vi "Camera.v7.vi"() -> ()   [LabVIEW 2015]
uses:
  Camera Properties.ctl
  Microscope Settings.ctl
  CameraState.ctl
  ModeEnum.ctl
  Stack_State.ctl
  Stack Track.ctl
  CameraControlTypeDef.ctl
  <vilib>/DAQmx/write.llb/DAQmx Write (Digital 1D Wfm NChan NSamp).vi
  <vilib>/DAQmx/write.llb/DAQmx Write (Analog 1D Wfm NChan NSamp).vi
  <vilib>/DAQmx/create/channels.llb/DAQmx Create Channel (DO-Digital Output).vi
  <vilib>/DAQmx/create/channels.llb/DAQmx Create Channel (AO-Voltage-Basic).vi
  <vilib>/Waveform/WDTOps.llb/WDT Number of Waveform Samples DBL.vi
  <vilib>/DAQmx/configure/timing.llb/DAQmx Timing (Sample Clock).vi
  <vilib>/Waveform/DWDTOps.llb/DWDT Uncompress Digital.vi
  <vilib>/DAQmx/miscellaneous.llb/DAQmx Fill In Error Info.vi
  <vilib>/vision/NI_Vision_Development_Module.lvlib
panel:
  out "Numeric 3":i32
  in  "Tab Control":enum32{"Camera Settings", "Recording"}(tab)
  in  "Microscope Settings":T1={"Mode"=enum."XY", {"Scanning Mode"=12.0, "Slit Width /%"=5.0}, "Piezo Position /um"=0.0, "Exposure/ms"=40.0, "Samples per millisecond"=100.0, "Relax/ms"=10.0, "Readout Direction"=2.0, "Trigger Source"=2.0, "Camera Delay"=11.0} {"Camera Delay" min=0.0 max=10.0 step=0.05; "Trigger Source" items=["Internal"=1.0, "External"=2.0]; "Readout Direction" items=["Forward"=1.0, "Backward"=2.0]; "?"."Scanning Mode" items=["Full Frame"=1.0, "Slit Scanning"=12.0]; "Piezo Position /um" min=0.0 max=10.0 step=0.1}
  in  "Scan":bool
  in  "Scan Continuously":bool
  out "error IO":errorcluster
  in  "V Height":dbl=2048.0 min=4.0 max=2048.0 step=4.0
  in  "V Offset":dbl min=0.0 max=0.0 step=4.0
  in  "H Offset":dbl min=0.0 max=0.0 step=4.0
  in  "H Width":dbl min=4.0 max=2048.0 step=4.0
  in  "Advanced DCAM Controls":i32(listbox) caption="Multicolumn Listbox"
  in  "Slit width":sgl
  in  "Properties":T2=4211904 items=["SENSOR MODE"=4212128, "CCD MODE"=4212384, "READOUT MODE"=4211872, "ACTIVE VIEW INDEX"=4343136, "BITS PER CHANNEL"=4342976, "IMAGE PIXEL TYPE"=4343296, "BINNING"=4215968, "EXPOSURE TIME"=2049184, "CONTRAST GAIN"=3163312, "CONTRAST OFFSET"=3163328, "LIGHT MODE"=2114720, "SENSITIVITY"=2114992, "PHOTON IMAGING MODE"=2115200, "HIGH DYNAMIC RANGE MODE"=3163360, "WHITE BALANCE"=3163568, "TEMPERATURE"=2115232, "TEMPERATURE TARGET"=2115264, "SENSOR COOLER FAN"=2115296, "LINEBUNDLE HEIGHT"=4212192, "MECHANICAL SHUTTER"=2115488, "BACK FOCUS POSITION"=8422304, "TRIGGER CONNECTOR"=1066432, "TRIGGER SOURCE"=1066144, "OUTPUT TRIGGER SOURCE"=1852576, "TRIGGER GLOBAL EXPOSURE"=2049680, "FIRST TRIGGER BEHAVIOR"=2049696, "CHANNEL SYNC"=1852352, "READOUT DIRECTION"=4211904, "PRE HSYNC COUNT"=1852704, "INTERNAL LINE SPEED"=4191408, "INTERNAL LINE INVERVAL"=4191424]
  out "Mixed Signal Graph":T3(graph)
  out "Image":T4(plugin-control)
  out "Histogram":T5(graph)
  in  "stop":bool
  in  "Signals Debugger":bool
  in  "Calibration":bool
  in  "MultiD Scan":bool
  in  "Stage Controller":bool
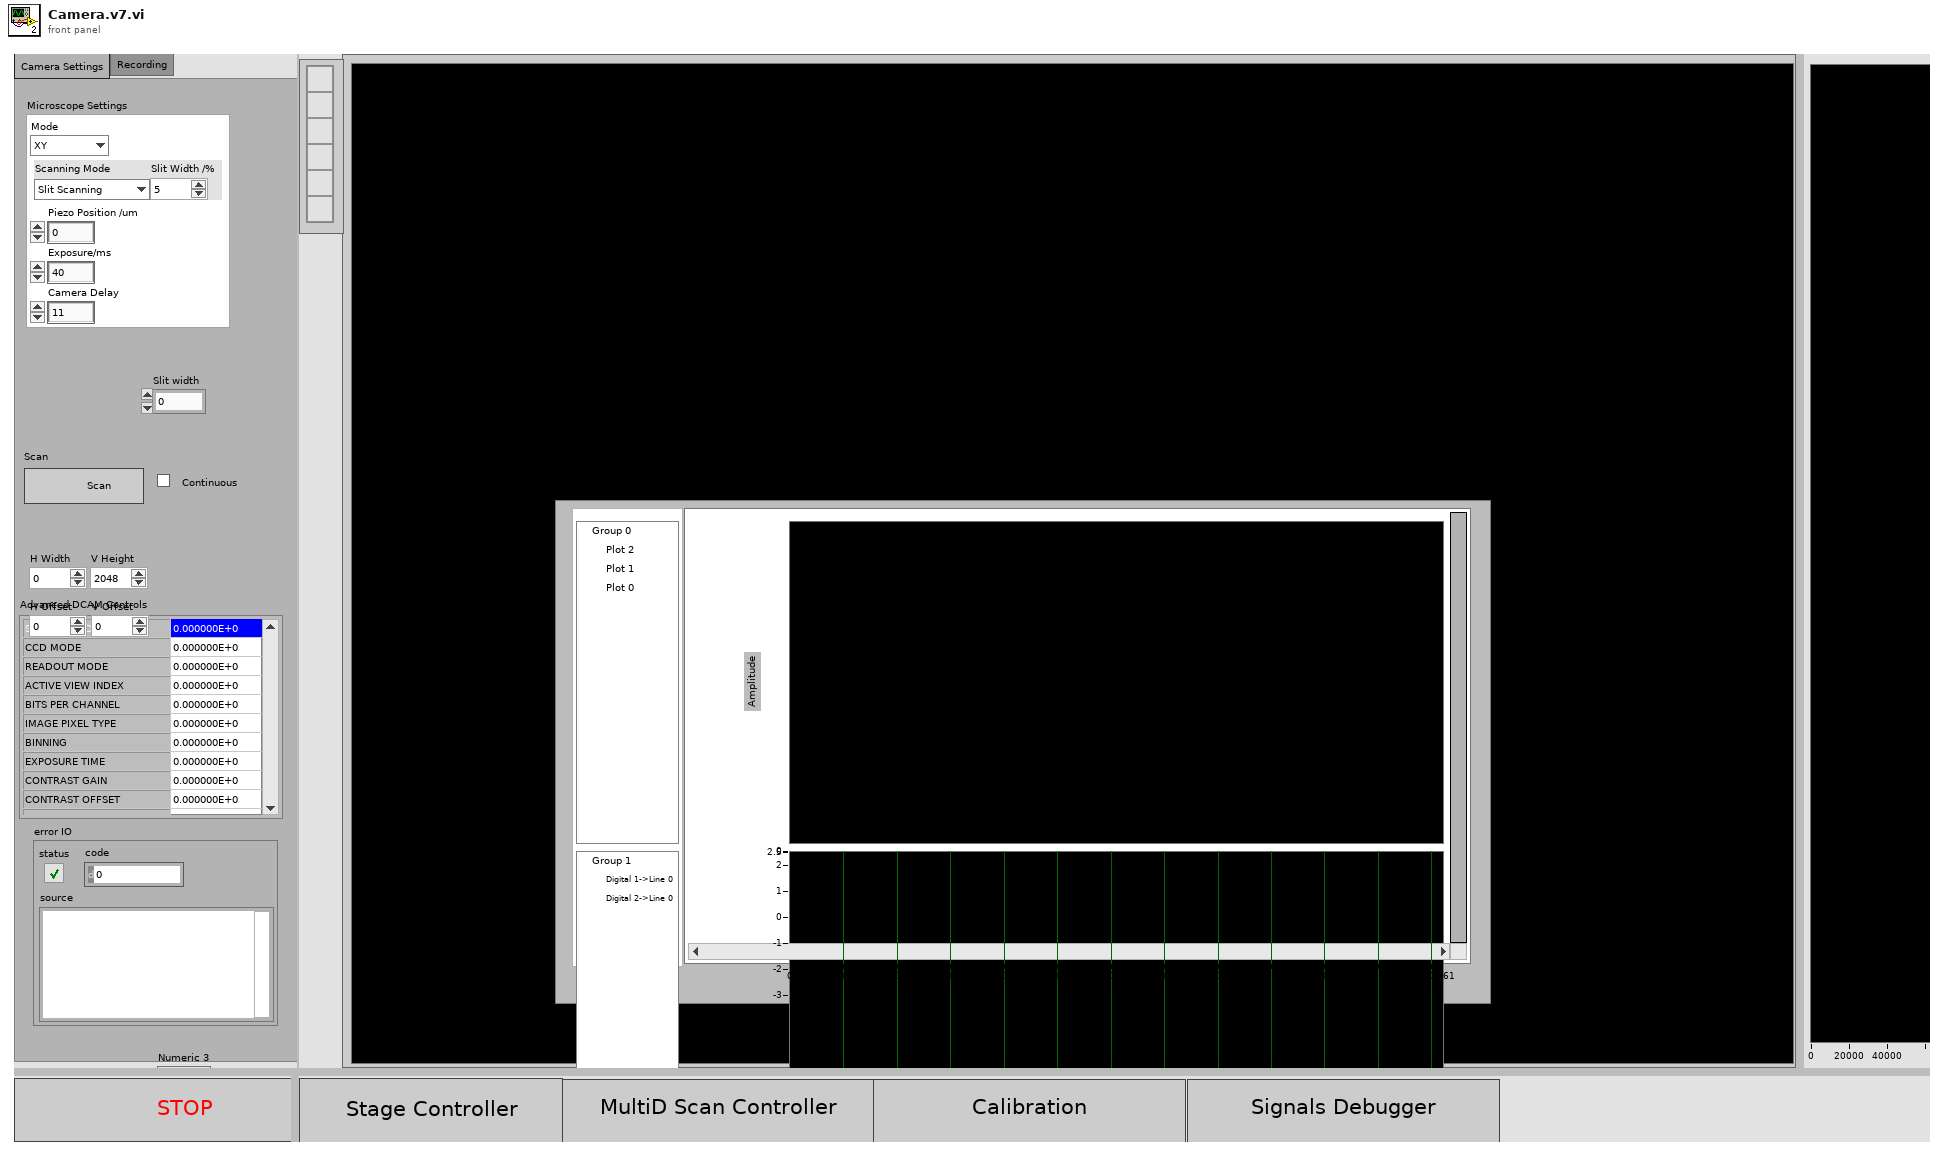
[diagram p1: front panel]
types:
  T1 = typedef "Microscope Settings.ctl" = cluster{"Mode":enum16{"X", "XY", "XYZ", "XYZT", "XYZC"}, cluster{"Scanning Mode":dbl, "Slit Width /%":dbl}, "Piezo Position /um":dbl, "Exposure/ms":dbl, "Samples per millisecond":dbl, "Relax/ms":dbl, "Readout Direction":dbl, "Trigger Source":dbl, "Camera Delay":dbl}
  T2 = typedef "Camera Properties.ctl" = u32
  T3 = cluster{waveform(dbl)[], "Digital Waveform":digitalwaveform, "Digital Waveform":digitalwaveform}
  T4 = typedef "IMAQ Image.ctl" = refnum<image>
  T5 = cluster{"Starting Value":sgl, "Incremental Value":sgl, "Histogram":u32[]}
  T6 = cluster{"height":u32, "width":u32, "datatype":u32}
  T7 = typedef "CameraState.ctl" = enum16{"init", "active", "deinit"}
  T8 = typedef "ModeEnum.ctl" = enum16{"Idle", "generateWaves", "runWaves", "stop"}
  T9 = cluster{"Mode":u32, "Polarity":u32, "Times":u32, "Delay":dbl}
  T10 = typedef "CameraControlTypeDef.ctl" = enum16{"Idle", "IntervalLineInt", "Ram Record", "HardDisk Record", "Disengage Update", "Update", "ROI", "Binning", "Scan Mode", "Trigger Mode", "Readout Mode", "Readout Direction", "Preview", "ROIWindow", "Trigger Source"}
  T11 = typedef "Stack_State.ctl" = cluster{"State":T12, "Stack Number":i32, "Image":u16[][], "Stacks":i32}
  T12 = typedef "Stack Track.ctl" = enum16{"Idle", "Display", "Start Sequence", "Read Disk", "STOP", "Collecting", "End"}
  T13 = typedef "Image Type" = u32
  T14 = cluster{"Value":i32, "Minimum":i32, "Maximum":i32, "Increment":i32}
  T15 = cluster{"State":T12, "Timeout":i32, "Data 16":u16[][], "Timeout":i32}
  T16 = cluster{"Enum":T10, "Trigger Source":dbl, "timeout in ms (-1)":i32}
  T17 = cluster{"Enum":T10, "Trigger Source":dbl, "Property ID":u32}
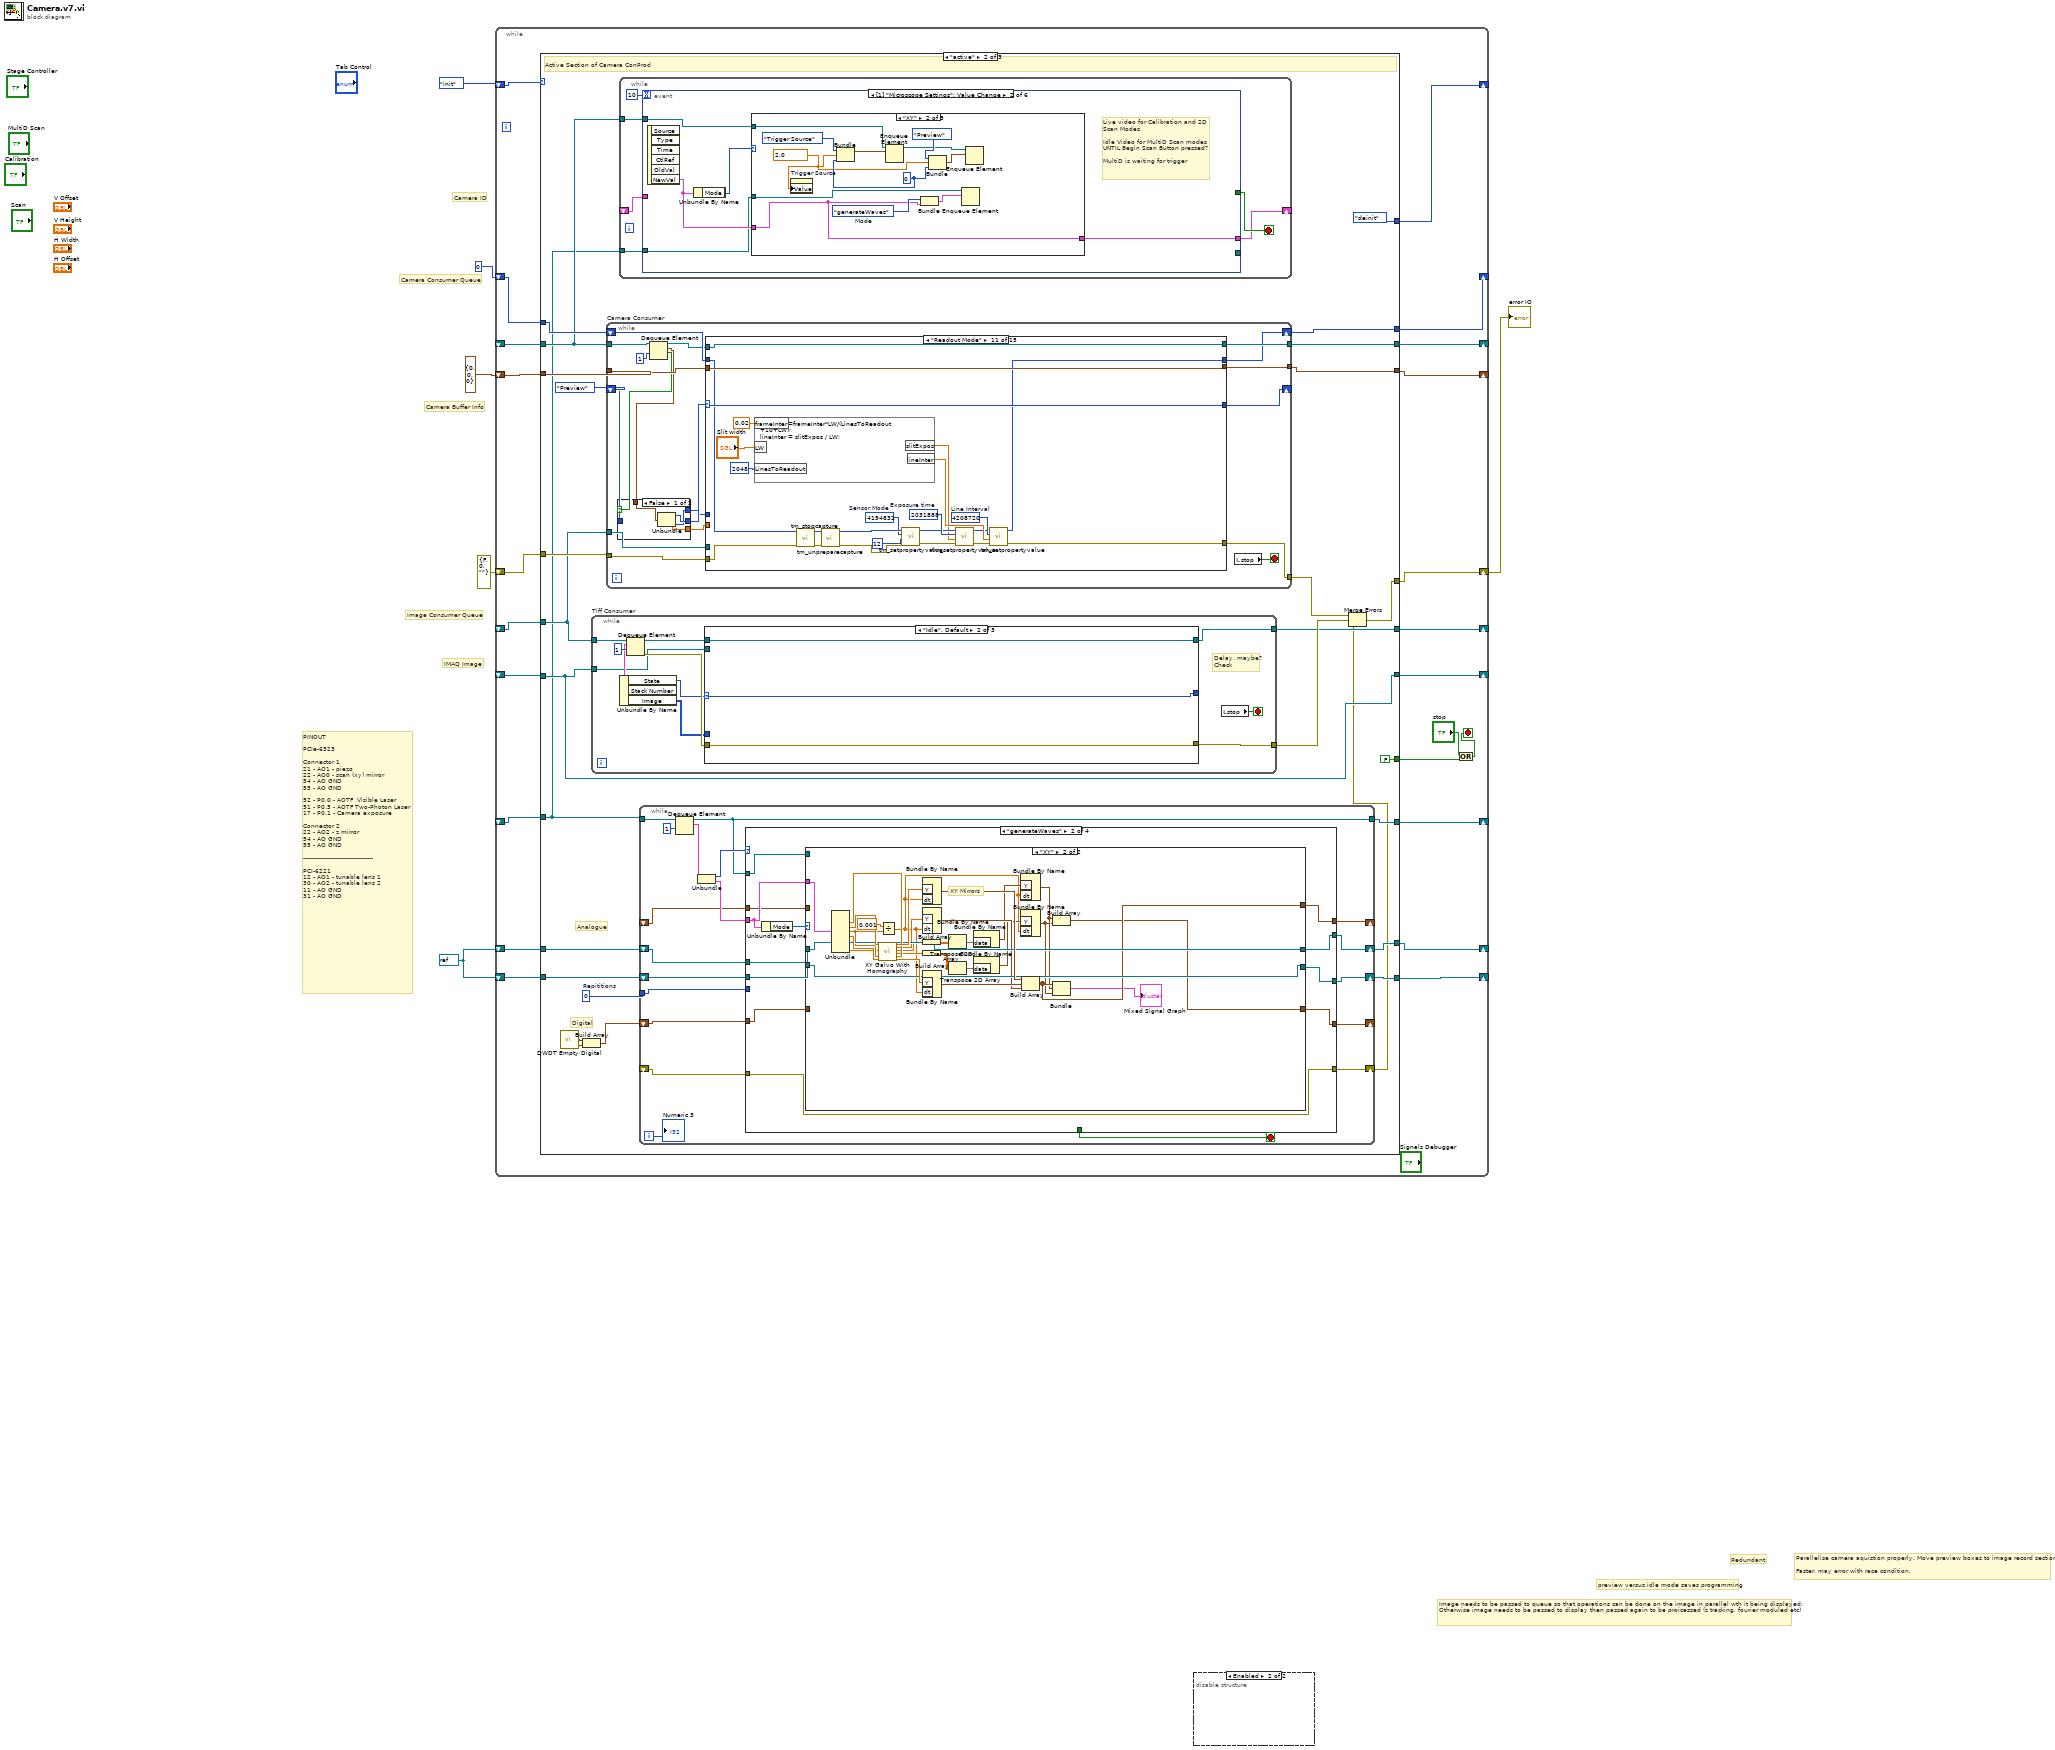
[diagram p0: block diagram]
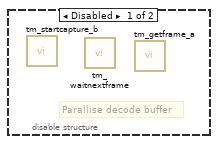
[diagram p2: hidden frame]
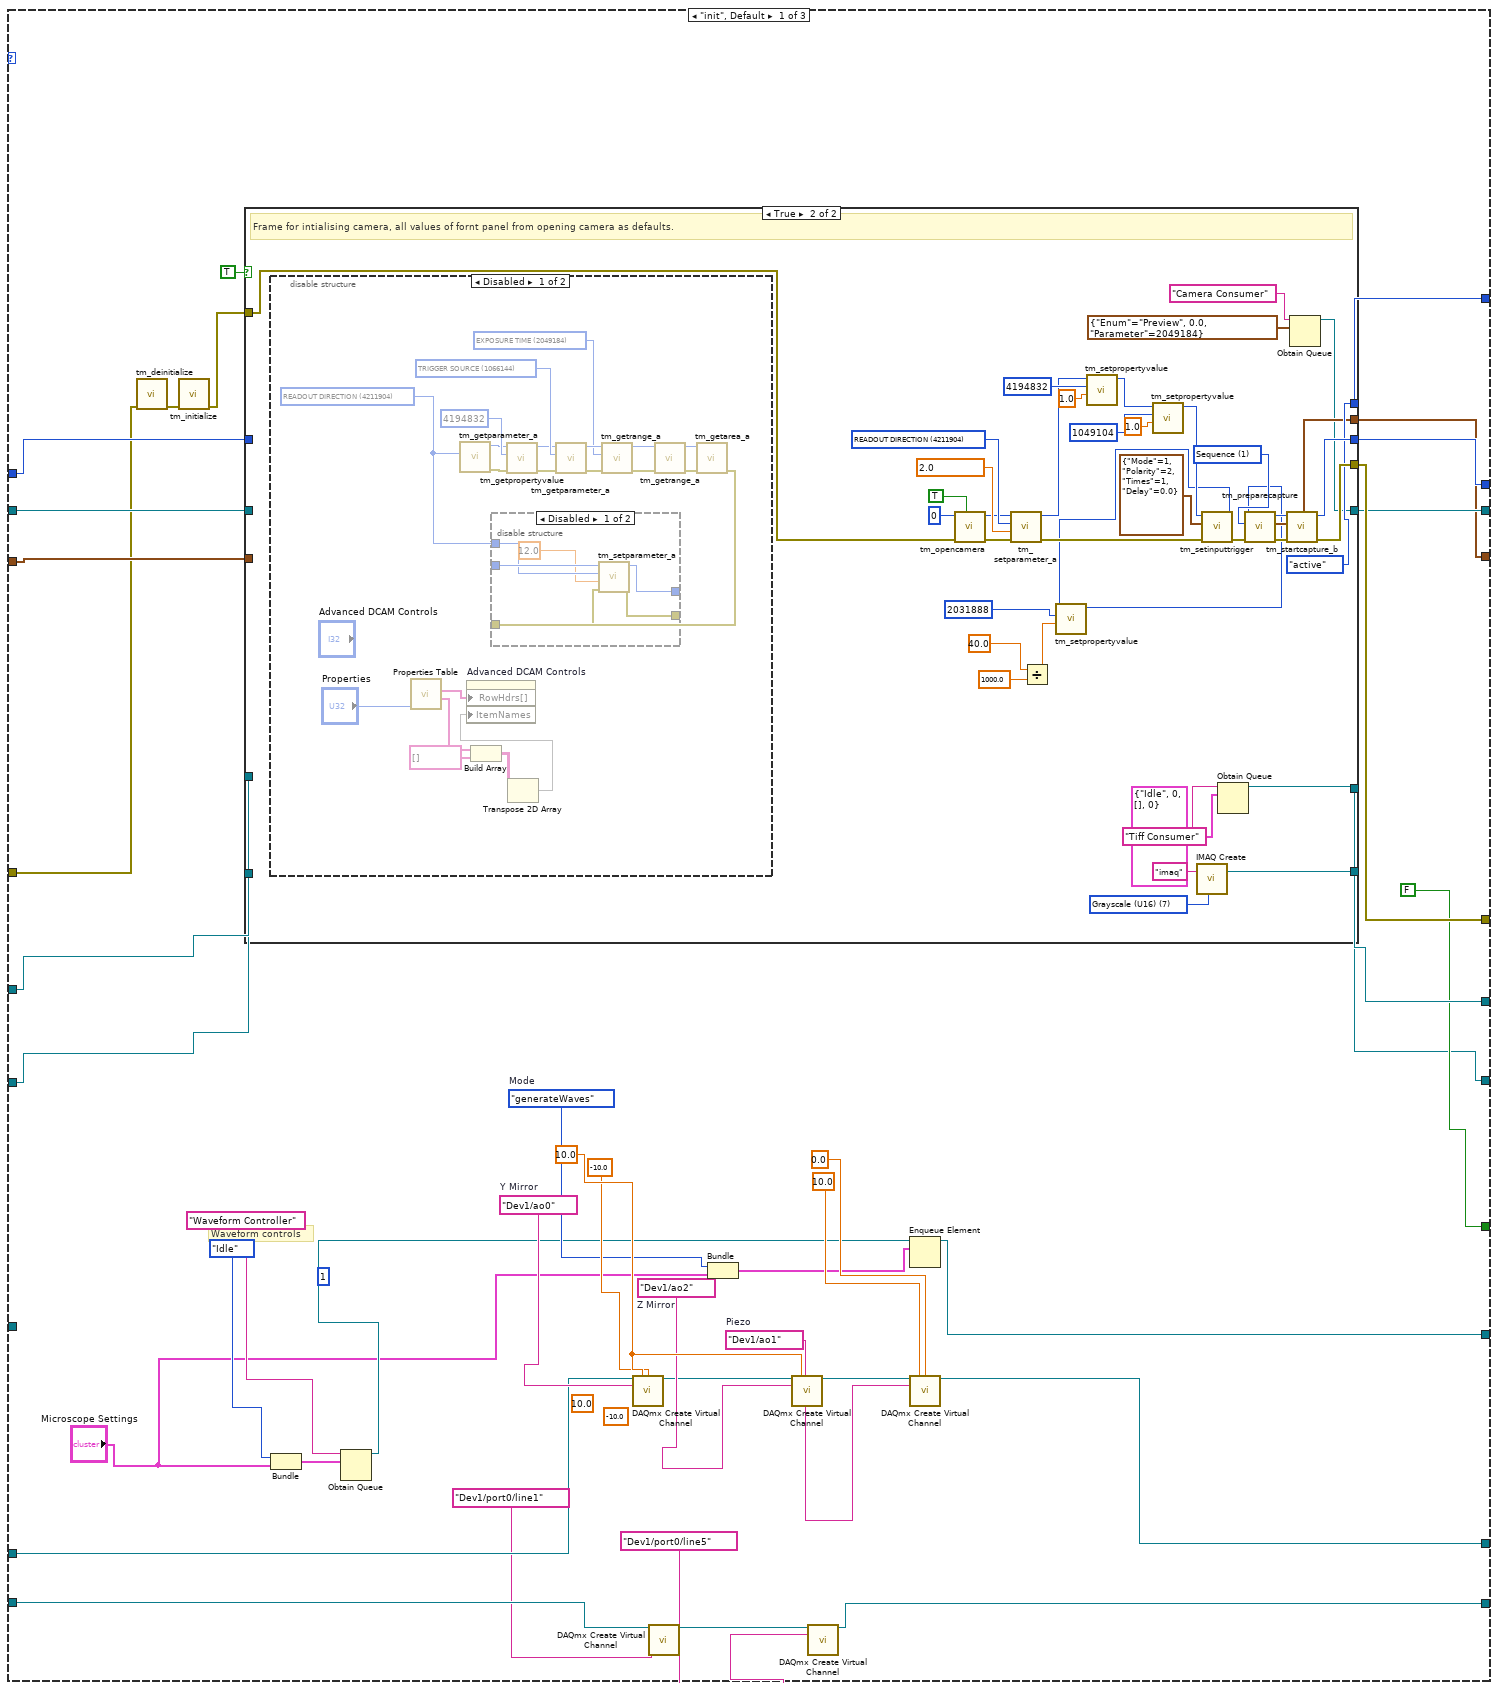
[diagram p3: hidden frame]
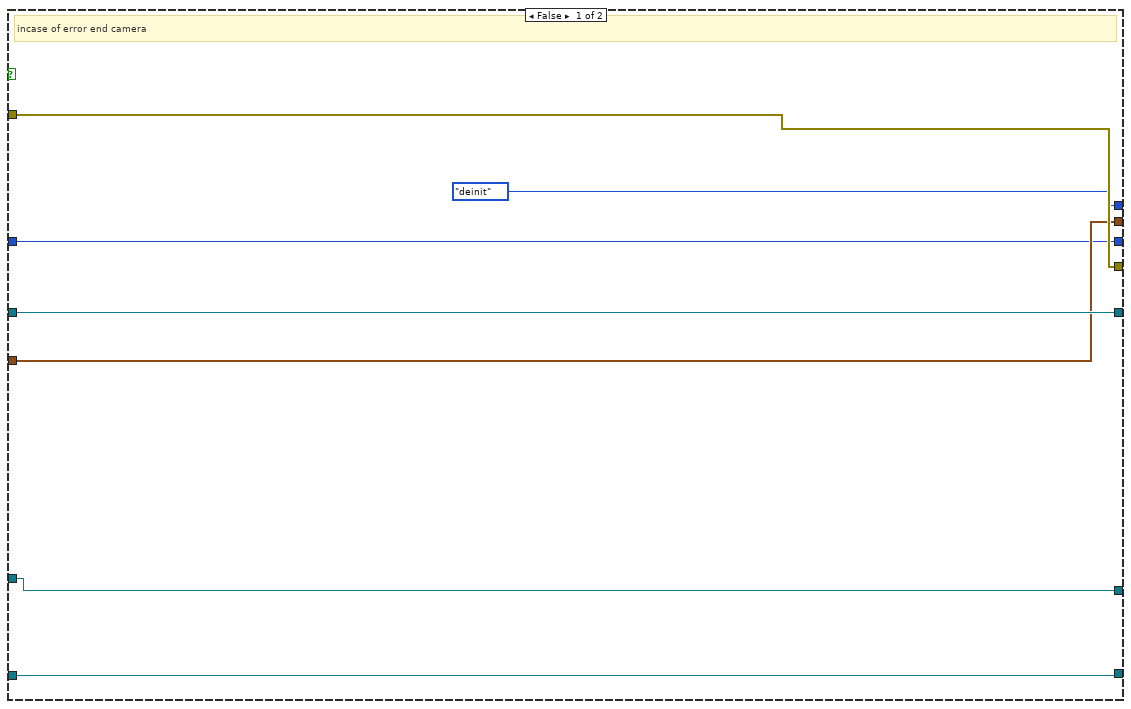
[diagram p4: hidden frame]
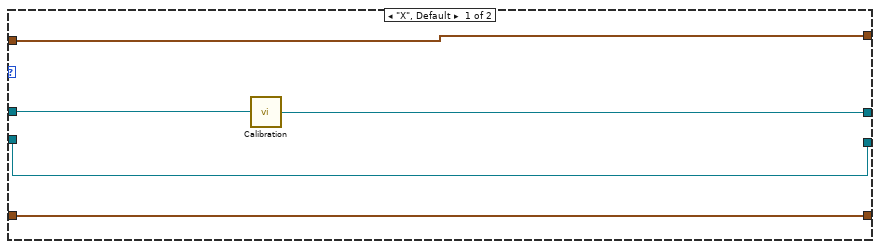
[diagram p8: hidden frame]
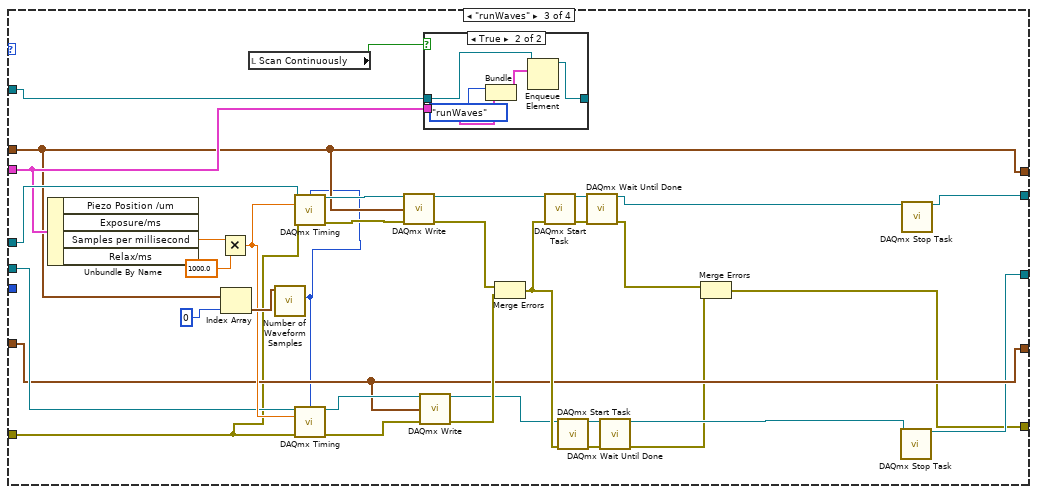
[diagram p9: hidden frame]
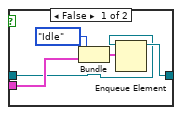
[diagram p10: hidden frame]
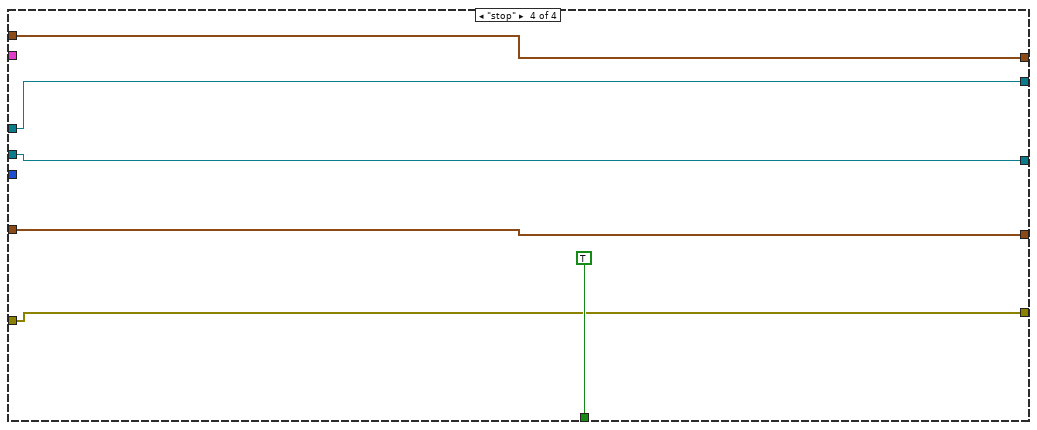
[diagram p11: hidden frame]
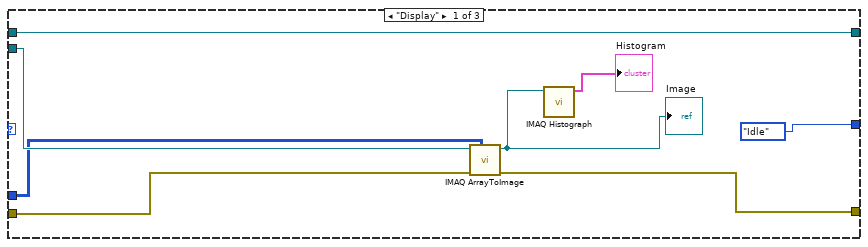
[diagram p12: hidden frame]
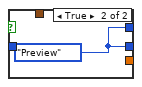
[diagram p14: hidden frame]
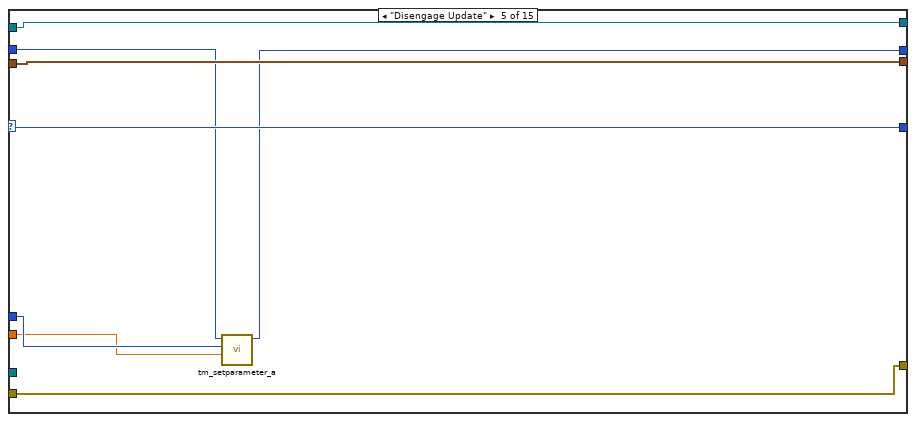
[diagram p19: hidden frame]
diagram:
  w3 = refnum<k21> refnum ("Mirror Z 2")
  # "PINOUT\n\nPCIe-6323\n\nConnector 1\n21 - AO1 - piezo\n22 - AO0 - scan (xy) mirror\n54 - AO GND\n55 - AO GND\n\n52 - P0.0 - AOTF  Visible Laser\n51 - P0.5 - AOTF Two-Photon Laser\n17 - P0.1 - Camera exposure\n\nConnector 2\n22 - AO2 - z mirror\n54 - AO GND\n55 - AO GND\n\n-----------------------------------\n\nPCI-6221\n12 - AO1 - tunable lens 1\n30 - AO2 - tunable lens 2\n11 - AO GND\n31 - AO GND"
  # "IMAQ Image"
  # "Camera Buffer Info"
  # "Image needs to be passed to queue so that operations can be done on the image in parallel wth it being displayed;\nOtherwise image needs to be passed to display then passed again to be proicessed (z tracking, fourier moduled etc)"
  # "preview versus idle mode saves programming"
  # "Parallelise camera aquistion properly. Move preview boxes to image record section.\n\nFaster. may error with race condition."
  # "Redundant"
  # "Image Consumer Queue"
  # "Camera Consumer Queue"
  # "Camera ID"
  n1 = while {
    shift-right: [w29] -> _
    shift-left: CameraState."init" -> [w28]
    shift-right: [w27] -> _
    shift-left: u32 0 ("Handle out") -> [w26]
    shift-right: [w25] -> w5
    shift-left: errorcluster {"status"=FALSE, "code"=0, "source"=""} ("error IO") -> [w24]
    shift-right: [w22] -> _
    shift-left: _ -> [w21]
    shift-right: [w23] -> _
    shift-left: _ -> [w20]
    shift-right: [w16] -> _
    shift-left: T6 {"height"=0, "width"=0, "datatype"=0} ("Buffer Info") -> [w15]
    shift-right: [w14] -> _
    shift-left: _ -> [w13]
    shift-right: [w12] -> _
    shift-left: w3 -> [w11]
    shift-right: [w9] -> _
    shift-left: w3 -> [w10]
    shift-right: [w8] -> _
    shift-left: _ -> [w7]
    stop <- w18 stop-if-true
    n2 = case shown="\"active\"" w28 {
      tunnel: [w68 CameraState."deinit" CameraState."init"] -> w29
      tunnel: [w67 w170 w561] -> w27
      tunnel: w26 -> [w45 w171 w561]
      tunnel: [w66 w169 w564] -> w25
      tunnel: w24 -> [w44 w163 w565]
      tunnel: [w65 w166 w548] -> w23
      tunnel: [w64 w165 w544] -> w22
      tunnel: w21 -> [w62 w158 w544]
      tunnel: w20 -> [w63 w156 w548]
      tunnel: [FALSE ("stop") FALSE ("stop") TRUE ("stop")] -> w17
      tunnel: [w60 w161 w558] -> w16
      tunnel: w15 -> [w59 w160 w558]
      tunnel: w13 -> [w57 w157 w557]
      tunnel: [w58 w157 w557] -> w14
      tunnel: w7 -> [_ w148 w543]
      tunnel: [w49 w149 w555] -> w12
      tunnel: w11 -> [w46 w152 w555]
      tunnel: w10 -> [w42 w151 w553]
      tunnel: [w33 w150 w553] -> w9
      tunnel: [w41 w147 w543] -> w8
      frame "init", Default {
        (unwired) 1 ("max queue size (-1, unlimited)")
        w39 = ModeEnum."generateWaves"  # Mode
        (unwired) -10.0 ("minimum value")
        (unwired) 10.0 ("maximum value")
        w52 = tag "Dev1/ao1"  # Piezo
        w53 = tag "Dev1/ao2"  # Z Mirror
        w54 = tag "Dev1/ao0"  # Y Mirror
        w56 = 10.0 ("maximum value")
        # "Waveform controls"
        n3 = call "tm_deinitialize.vi"("error in (no error)"=w44) -> ("error out"=w70:errorcluster)  [unwired: 10 in]
        n4 = call "tm_initialize.vi"("error in (no error)"=w70) -> ("error out"=w69:errorcluster)  [unwired: 7 in, 3 out]
        n5 = case shown="True" TRUE {
          tunnel: w69 -> [w77 w114]
          tunnel: [CameraState."deinit" CameraState."active"] -> w68
          tunnel: [w77 w111] -> w66
          tunnel: [w72 w109] -> w67
          tunnel: [w75 w98] -> w65
          tunnel: [w74 w106] -> w64
          tunnel: w63 -> [w75 _]
          tunnel: w62 -> [w74 _]
          tunnel: [w73 w104] -> w60
          tunnel: w59 -> [w73 _]
          tunnel: w45 -> [w72 _]
          tunnel: [w71 w101] -> w58
          tunnel: w57 -> [w71 _]
          frame False {
            # "incase of error end camera"
          }
          frame True {
            w96 = sgl 2.0 items=["Forward"=1.0, "Backward"=2.0] ("Readout Direction")
            w97 = u32 4211904 items=["SENSOR MODE"=4212128, "CCD MODE"=4212384, "READOUT MODE"=4211872, "ACTIVE VIEW INDEX"=4343136, "BITS PER CHANNEL"=4342976, "IMAGE PIXEL TYPE"=4343296, "BINNING"=4215968, "EXPOSURE TIME"=2049184, "CONTRAST GAIN"=3163312, "CONTRAST OFFSET"=3163328, "LIGHT MODE"=2114720, "SENSITIVITY"=2114992, "PHOTON IMAGING MODE"=2115200, "HIGH DYNAMIC RANGE MODE"=3163360, "WHITE BALANCE"=3163568, "TEMPERATURE"=2115232, "TEMPERATURE TARGET"=2115264, "SENSOR COOLER FAN"=2115296, "LINEBUNDLE HEIGHT"=4212192, "MECHANICAL SHUTTER"=2115488, "BACK FOCUS POSITION"=8422304, "TRIGGER CONNECTOR"=1066432, "TRIGGER SOURCE"=1066144, "OUTPUT TRIGGER SOURCE"=1852576, "TRIGGER GLOBAL EXPOSURE"=2049680, "FIRST TRIGGER BEHAVIOR"=2049696, "CHANNEL SYNC"=1852352, "READOUT DIRECTION"=4211904, "PRE HSYNC COUNT"=1852704, "INTERNAL LINE SPEED"=4226000, "INTERNAL LINE INTERVAL"=4226016] ("Parameter")
            w103 = T13 7 items=["Grayscale (U8)", "Grayscale (I16)", "Grayscale (SGL)", "Complex (CSG)", "RGB (U32)", "HSL (U32)", "RGB (U64)", "Grayscale (U16)"] ("Image Type")
            w113 = 1 items=["Snap", "Sequence"] ("Capture mode")
            # "Frame for intialising camera, all values of fornt panel from opening camera as defaults."
            n6 = disable-structure shown="Disabled" {
              frame Disabled {
                w135 = u32 2049184 items=["SENSOR MODE"=4212128, "CCD MODE"=4212384, "READOUT MODE"=4211872, "ACTIVE VIEW INDEX"=4343136, "BITS PER CHANNEL"=4342976, "IMAGE PIXEL TYPE"=4343296, "BINNING"=4215968, "EXPOSURE TIME"=2049184, "CONTRAST GAIN"=3163312, "CONTRAST OFFSET"=3163328, "LIGHT MODE"=2114720, "SENSITIVITY"=2114992, "PHOTON IMAGING MODE"=2115200, "HIGH DYNAMIC RANGE MODE"=3163360, "WHITE BALANCE"=3163568, "TEMPERATURE"=2115232, "TEMPERATURE TARGET"=2115264, "SENSOR COOLER FAN"=2115296, "LINEBUNDLE HEIGHT"=4212192, "MECHANICAL SHUTTER"=2115488, "BACK FOCUS POSITION"=8422304, "TRIGGER CONNECTOR"=1066432, "TRIGGER SOURCE"=1066144, "OUTPUT TRIGGER SOURCE"=1852576, "TRIGGER GLOBAL EXPOSURE"=2049680, "FIRST TRIGGER BEHAVIOR"=2049696, "CHANNEL SYNC"=1852352, "READOUT DIRECTION"=4211904, "PRE HSYNC COUNT"=1852704, "INTERNAL LINE SPEED"=4191408, "INTERNAL LINE INVERVAL"=4191424] ("Parameter")
                w118 = T2 4211904 items=["SENSOR MODE"=4212128, "CCD MODE"=4212384, "READOUT MODE"=4211872, "ACTIVE VIEW INDEX"=4343136, "BITS PER CHANNEL"=4342976, "IMAGE PIXEL TYPE"=4343296, "BINNING"=4215968, "EXPOSURE TIME"=2049184, "CONTRAST GAIN"=3163312, "CONTRAST OFFSET"=3163328, "LIGHT MODE"=2114720, "SENSITIVITY"=2114992, "PHOTON IMAGING MODE"=2115200, "HIGH DYNAMIC RANGE MODE"=3163360, "WHITE BALANCE"=3163568, "TEMPERATURE"=2115232, "TEMPERATURE TARGET"=2115264, "SENSOR COOLER FAN"=2115296, "LINEBUNDLE HEIGHT"=4212192, "MECHANICAL SHUTTER"=2115488, "BACK FOCUS POSITION"=8422304, "TRIGGER CONNECTOR"=1066432, "TRIGGER SOURCE"=1066144, "OUTPUT TRIGGER SOURCE"=1852576, "TRIGGER GLOBAL EXPOSURE"=2049680, "FIRST TRIGGER BEHAVIOR"=2049696, "CHANNEL SYNC"=1852352, "READOUT DIRECTION"=4211904, "PRE HSYNC COUNT"=1852704, "INTERNAL LINE SPEED"=4191408, "INTERNAL LINE INVERVAL"=4191424] ("Parameter")
                w138 = u32 1066144 items=["SENSOR MODE"=4212128, "CCD MODE"=4212384, "READOUT MODE"=4211872, "ACTIVE VIEW INDEX"=4343136, "BITS PER CHANNEL"=4342976, "IMAGE PIXEL TYPE"=4343296, "BINNING"=4215968, "EXPOSURE TIME"=2049184, "CONTRAST GAIN"=3163312, "CONTRAST OFFSET"=3163328, "LIGHT MODE"=2114720, "SENSITIVITY"=2114992, "PHOTON IMAGING MODE"=2115200, "HIGH DYNAMIC RANGE MODE"=3163360, "WHITE BALANCE"=3163568, "TEMPERATURE"=2115232, "TEMPERATURE TARGET"=2115264, "SENSOR COOLER FAN"=2115296, "LINEBUNDLE HEIGHT"=4212192, "MECHANICAL SHUTTER"=2115488, "BACK FOCUS POSITION"=8422304, "TRIGGER CONNECTOR"=1066432, "TRIGGER SOURCE"=1066144, "OUTPUT TRIGGER SOURCE"=1852576, "TRIGGER GLOBAL EXPOSURE"=2049680, "FIRST TRIGGER BEHAVIOR"=2049696, "CHANNEL SYNC"=1852352, "READOUT DIRECTION"=4211904, "PRE HSYNC COUNT"=1852704, "INTERNAL LINE SPEED"=4191408, "INTERNAL LINE INVERVAL"=4191424] ("Parameter")
                n7 = call "Properties Table.vi"("Properties"="Properties") -> ("Value Stirngs Out"=w123:string[], "Row Headers"=w124:string[])  [unwired: 4 in, 2 out]
                n8 = call "tm_getparameter_a.vi"("Parameter"=w118) -> ("error out"=w127:errorcluster, "Handle out"=w129:u32)  [unwired: 8 in, 1 out]
                n9 = Build Array(w123, string[] [] ("element")) -> (w121:string[][])
                n10 = call "tm_getpropertyvalue.vi"("error in (no error)"=w127, "Property ID"=u32 4194832, "Handle in"=w129) -> ("error out"=w128:errorcluster, "Handle out"=w117:u32)  [unwired: 6 in, 1 out]
                n11 = Transpose 2D Array(2D array=w121) -> (transposed array=w120:string[][])
                n12 = property on="Advanced DCAM Controls" class="MCListbox (strict)"("RowHdrs[]"=w124, "ItemNames"=w120) -> ()  [unwired: 2 in, 2 out]
                n13 = call "tm_getparameter_a.vi"("error in (no error)"=w128, "Parameter"=w138, "Handle in"=w117) -> ("error out"=w136:errorcluster, "Handle out"=w137:u32)  [unwired: 6 in, 1 out]
                n14 = call "tm_getrange_a.vi"("error in (no error)"=w136, "Parameter"=w135, "Handle in"=w137) -> ("error out"=w133:errorcluster, "Handle out"=w134:u32)  [unwired: 2 in, 5 out]
                n15 = call "tm_getrange_a.vi"("error in (no error)"=w133, "Handle in"=w134) -> ("error out"=w132:errorcluster, "Handle out"=w131:u32)  [unwired: 3 in, 5 out]
                n16 = call "tm_getarea_a.vi"("error in (no error)"=w132, "Handle in"=w131) -> ("error out"=w119:errorcluster, "H Offset"=w126:T14)  [unwired: 4 in, 4 out]
                n17 = disable-structure shown="Disabled" {
                  disable-tunnel: _ -> [w144 _]
                  disable-tunnel: [w143 _] -> _
                  disable-tunnel: w119 -> [w142 w145]
                  disable-tunnel: [w141 w145] -> _
                  disable-tunnel: w118 -> [w140 _]
                  frame Disabled {
                    n18 = call "tm_setparameter_a.vi"("error in (no error)"=w142, "Value in"=12.0, "Parameter"=w140, "Handle in"=w144) -> ("error out"=w141:errorcluster, "Handle out"=w143:u32)  [unwired: 6 in]
                  }
                  frame Enabled {
                  }
                }
              }
              frame Enabled {
              }
            }
            n19 = call "tm_opencamera.vi"("Force Open"=TRUE, "error in (no error)"=w114, "Camera Index"=u32 0) -> ("error out"=w94:errorcluster, "Handle out"=w95:u32)  [unwired: 6 in, 1 out]
            n20 = call "tm_setparameter_a.vi"("error in (no error)"=w94, "Value in"=w96, "Parameter"=w97, "Handle in"=w95) -> ("error out"=w85:errorcluster, "Handle out"=w84:u32)  [unwired: 6 in]
            n21 = Divide(x=sgl 40.0 ("Value in"), y=sgl 1000.0) -> (x/y=w78:sgl)
            n22 = call "tm_setpropertyvalue.vi"("Value in"=sgl 1.0, "Property ID"=u32 4194832, "Handle in"=w84) -> ("Handle out"=w88:u32)  [unwired: 7 in, 1 out]
            n23 = call "tm_setpropertyvalue.vi"("Value in"=sgl 1.0, "Property ID"=u32 1049104, "Handle in"=w88) -> ("Handle out"=w86:u32)  [unwired: 7 in, 1 out]
            n24 = call "IMAQ Create"("Image Name"="imaq", "Image Type"=w103) -> ("New Image"=w101:T4)  [unwired: 3 in, 1 out]
            n25 = call <userlib>:"tm_setinputtrigger.vi"("error in (no error)"=w85, "Parameters"=T9 {"Mode"=1, "Polarity"=2, "Times"=1, "Delay"=0.0}, "Handle in"=w86) -> ("error out"=w93:errorcluster, "Handle out"=w82:u32)  [unwired: 7 in]
            n26 = call "tm_setpropertyvalue.vi"("Value in"=w78, "Property ID"=u32 2031888, "Handle in"=w82) -> ("Handle out"=w81:u32)  [unwired: 7 in, 1 out]
            n27 = Obtain Queue(name (unnamed)="Tiff Consumer", element data type=T11 {"State"=enum."Idle", "Stack Number"=0, "Image"=[], "Stacks"=0} ("input cluster")) -> (queue out=w106:refnum<queue>)  [unwired: 3 in, 2 out]
            n28 = call "tm_preparecapture.vi"("error in (no error)"=w93, "Capture mode"=w113, "Handle in"=w81) -> ("error out"=w112:errorcluster, "Buffer Info"=w104:T6, "Handle out"=w110:u32)  [unwired: 5 in, 1 out]
            n29 = call "tm_startcapture_b.vi"("error in (no error)"=w112, "Handle in"=w110) -> ("error out"=w111:errorcluster, "Handle out"=w109:u32)  [unwired: 8 in]
            n30 = Obtain Queue(name (unnamed)="Camera Consumer", element data type=cluster{"Enum":T10, dbl, "Parameter":u32} {"Enum"=enum."Preview", 0.0, "Parameter"=2049184}) -> (queue out=w98:refnum<queue>)  [unwired: 3 in, 2 out]
          }
        }
        n31 = Bundle("Mode"=ModeEnum."Idle", "Microscope Settings"="Microscope Settings") -> (w36:cluster{"Mode":T8, "Microscope Settings":T1})  [unwired: 1 in]
        n32 = Obtain Queue(name (unnamed)="Waveform Controller", element data type=w36) -> (queue out=w35:refnum<queue>)  [unwired: 3 in, 2 out]
        n33 = call-poly <vilib>:"DAQmx Create Virtual Channel.vi"("task in"=w46, "maximum value"=w56, "minimum value"=-10.0, "physical channels"=w54) -> ("task out"=w48:refnum<k21>)  [unwired: 10 in, 1 out]
        n34 = call-poly <vilib>:"DAQmx Create Virtual Channel.vi"("task in"=w42, "lines"=tag "Dev1/port0/line1") -> ("task out"=w43:refnum<k21>)  [unwired: 12 in, 1 out]
        n35 = Bundle("Mode"=w39, "Microscope Settings"="Microscope Settings") -> (w40:cluster{"Mode":T8, "Microscope Settings":T1})  [unwired: 1 in]
        n36 = call-poly <vilib>:"DAQmx Create Virtual Channel.vi"("task in"=w48, "maximum value"=w56, "physical channels"=w53) -> ("task out"=w47:refnum<k21>)  [unwired: 11 in, 1 out]
        n37 = call-poly <vilib>:"DAQmx Create Virtual Channel.vi"("task in"=w43, "lines"=tag "Dev1/port0/line5") -> ("task out"=w33:refnum<k21>)  [unwired: 12 in, 1 out]
        n38 = Enqueue Element(queue=w35, element=w40) -> (queue out=w41:refnum<queue>)  [unwired: 2 in, 2 out]
        n39 = call-poly <vilib>:"DAQmx Create Virtual Channel.vi"("task in"=w47, "maximum value"=10.0 ("minimum value"), "minimum value"=0.0 ("maximum value"), "physical channels"=w52) -> ("task out"=w49:refnum<k21>)  [unwired: 10 in, 1 out]
      }
      frame "active" {
        w155 = 0  # Repititions
        # "Digital"
        # "Analogue"
        # "Active Section of Camera ConProd"
        n40 = call <vilib>:"DWDT Empty Digital.vi"() -> ("digital waveform out"=w153:digitalwaveform)  [unwired: 5 in]
        n41 = Build Array(w153, w153) -> (w154:digitalwaveform[])
        n42 = while "Tiff Consumer" {
          tunnel: [w295] -> w168
          tunnel: [w298] -> w165
          tunnel: w158 -> [w300]
          tunnel: w157 -> [w292]
          stop <- w302 stop-if-true
          # "Delay, maybe?\nCheck"
          n43 = Dequeue Element(queue=w300, timeout in ms (-1)=1) -> (queue out=w297:refnum<queue>, element=w299:T11, error out=w296:errorcluster)  [unwired: 1 in, 1 out]
          n44 = Unbundle By Name(w299) -> ("State"=w293:T12, "Image"=w294:u16[][])  [unwired: 1 out]
          n45 = case shown="\"Idle\", Default" w293 {
            selector: w293 -> [_ w313 w314]
            tunnel: [w310 w312 w315] -> w298
            tunnel: w297 -> [w310 w312 w315]
            tunnel: [Stack_Track."Idle" ("State") w313 w314] -> _
            tunnel: w294 -> [w305 _ _]
            tunnel: w292 -> [w309 _ _]
            tunnel: w296 -> [w308 w311 w316]
            tunnel: [w307 w311 w316] -> w295
            frame "Display" {
              n46 = call "IMAQ ArrayToImage"("Image Pixels (U16)"=w305, "error in (no error)"=w308, "Image"=w309) -> ("error out"=w307:errorcluster, "Image Out"=w304:T4)  [unwired: 7 in]
              "Image" <- w304
              n47 = call "IMAQ Histograph"("Image"=w304) -> ("Histogram Graph"=→"Histogram":T5)  [unwired: 7 in, 3 out]
            }
            frame "Idle", Default {
            }
            frame "Start Sequence" {
            }
          }
          n48 = local read "stop"() -> (w302:bool)
        }
        n49 = while "Camera Consumer" {
          tunnel: w163 -> [w334]
          tunnel: [w318] -> w167
          tunnel: w156 -> [w327]
          tunnel: [w335] -> w166
          shift-right: [w333] -> _
          shift-left: CameraControlTypeDef."Preview" ("Enum") -> [w323]
          tunnel: [w330] -> w161
          tunnel: w160 -> [w329]
          tunnel: w158 -> [w322]
          shift-right: [w331] -> w170
          shift-left: w171 -> [w332]
          stop <- w317 stop-if-true
          n50 = Dequeue Element(queue=w327, timeout in ms (-1)=1) -> (queue out=w326:refnum<queue>, element=w321:cluster{"Enum":T10, dbl, "Parameter":u32}, timed out?=w325:bool)  [unwired: 1 in, 1 out]
          n51 = case shown="False" w325 {
            tunnel: [w338 w340] -> w324
            tunnel: w323 -> [_ _]
            tunnel: w321 -> [w339 _]
            tunnel: [w337 _] -> w320
            tunnel: [w336 w340] -> w319
            frame False {
              n52 = Unbundle(w339) -> ("Enum"=w338:T10, w337:dbl, "Parameter"=w336:u32)
            }
            frame True {
              w340 = CameraControlTypeDef."Preview" ("Enum")
            }
          }
          n53 = case shown="\"Readout Mode\"" w324 {
            selector: w324 -> [w344 w349 w354 w359 w367 w372 w377 w382 w387 w392 w416 w422 _ w451 _]
            tunnel: w326 -> [w343 w350 w355 w360 w368 w373 w378 w383 w388 w393 w417 w418 w433 w453 w471]
            tunnel: [w343 w350 w355 w360 w368 w373 w378 w383 w388 w393 w417 w418 w433 w453 w471] -> w335
            tunnel: w334 -> [w345 w348 w353 w358 w366 w371 w376 w381 w386 w391 w396 w421 w425 w450 w462]
            tunnel: [w345 w348 w353 w358 w366 w371 w376 w381 w386 w391 w395 w421 w424 w450 w463] -> w318
            tunnel: [w344 w349 w354 w359 w367 w372 w377 w382 w387 w392 w416 w422 CameraControlTypeDef."Preview" ("Enum") w451 CameraControlTypeDef."Preview" ("Enum")] -> w333
            tunnel: w332 -> [w342 w347 w352 w357 w364 w370 w375 w380 w385 w390 w403 w420 w431 w452 w465]
            tunnel: [w342 w347 w352 w357 w363 w370 w375 w380 w385 w390 w410 w420 w429 w452 w464] -> w331
            tunnel: [w341 w346 w351 w356 w365 w369 w374 w379 w384 w389 w415 w419 w427 w449 w466] -> w330
            tunnel: w329 -> [w341 w346 w351 w356 w365 w369 w374 w379 w384 w389 w415 w419 w427 w449 _]
            tunnel: w322 -> [_ _ _ _ _ _ _ _ _ _ _ _ w426 _ _]
            tunnel: w320 -> [_ _ _ _ w361 _ _ _ _ _ _ _ _ _ w456]
            tunnel: w319 -> [_ _ _ _ w362 _ _ _ _ _ _ _ _ _ _]
            frame "Idle" {
            }
            frame "IntervalLineInt" {
            }
            frame "Ram Record" {
            }
            frame "HardDisk Record" {
            }
            frame "Disengage Update" {
              n54 = call "tm_setparameter_a.vi"("Value in"=w361, "Parameter"=w362, "Handle in"=w364) -> ("Handle out"=w363:u32)  [unwired: 7 in, 1 out]
            }
            frame "Update", Default {
            }
            frame "ROI" {
            }
            frame "Binning" {
            }
            frame "Scan Mode" {
            }
            frame "Trigger Mode" {
            }
            frame "Readout Mode" {
              w400 = u32 4194832  # Sensor Mode
              w411 = u32 2031888  # Exposure time
              w413 = u32 4208720  # Line Interval
              n55 = formula code="slitExpos=frameInter*LW/(LinesToReadout\n+10+LW);\nlineInter = slitExpos / LW;"("frameInter"=0.02 ("input variable"), "LW"="Slit width", "LinesToReadout"=2048 ("input variable")) -> ("slitExpos"=w407:dbl, "lineInter"=w412:dbl)
              n56 = call "tm_stopcapture.vi"("error in (no error)"=w396, "Handle in"=w403) -> ("error out"=w404:errorcluster, "Handle out"=w401:u32)  [unwired: 8 in]
              n57 = call "tm_unpreparecapture.vi"("error in (no error)"=w404, "Handle in"=w401) -> ("error out"=w397:errorcluster, "Handle out"=w402:u32)  [unwired: 8 in]
              n58 = call "tm_setpropertyvalue.vi"("error in (no error)"=w397, "Value in"=u32 12 ("Property ID"), "Property ID"=w400, "Handle in"=w402) -> ("error out"=w406:errorcluster, "Handle out"=w409:u32)  [unwired: 6 in]
              n59 = call "tm_setpropertyvalue.vi"("error in (no error)"=w406, "Value in"=w407, "Property ID"=w411, "Handle in"=w409) -> ("error out"=w405:errorcluster, "Handle out"=w408:u32)  [unwired: 6 in]
              n60 = call "tm_setpropertyvalue.vi"("error in (no error)"=w405, "Value in"=w412, "Property ID"=w413, "Handle in"=w408) -> ("error out"=w395:errorcluster, "Handle out"=w410:u32)  [unwired: 6 in]
            }
            frame "Readout Direction" {
            }
            frame "Preview" {
              n61 = call "tm_waitnextframe.vi"("error in (no error)"=w425, "Timeout"=500, "Handle in"=w431) -> ("error out"=w423:errorcluster, "Handle out"=w430:u32)  [unwired: 5 in, 2 out]
              n62 = case shown="No Error" w423 {
                selector: w423 -> [w434 w448]
                tunnel: w430 -> [w446 w447]
                tunnel: [w445 w447] -> w429
                tunnel: w427 -> [w444 _]
                tunnel: w426 -> [w443 _]
                tunnel: w425 -> [w438 _]
                tunnel: [w435 w448] -> w424
                frame No Error {
                  w440 = 0 ("Timeout")
                  n63 = call "tm_getframe_a.vi"("error in (no error)"=w434, "Buffer Info"=w444, "Handle in"=w446) -> ("error out"=w436:errorcluster, "Data 16"=w441:u16[][], "Handle out"=w445:u32)  [unwired: 4 in, 2 out]
                  n64 = Bundle("State"=Stack_Track."Display", "Timeout"=w440, "Data 16"=w441, "Timeout"=w440) -> (w439:T15)  [unwired: 1 in]
                  n65 = Enqueue Element(queue=w443, element=w439, error in (no error)=w438) -> (error out=w437:errorcluster)  [unwired: 1 in, 2 out]
                  n66 = Merge Errors(w436, w437) -> (w435:errorcluster)
                }
                frame Error {
                }
              }
            }
            frame "ROIWindow" {
            }
            frame "Trigger Source" {
              (unwired) u32 1066144 items=["SENSOR MODE"=4212128, "CCD MODE"=4212384, "READOUT MODE"=4211872, "ACTIVE VIEW INDEX"=4343136, "BITS PER CHANNEL"=4342976, "IMAGE PIXEL TYPE"=4343296, "BINNING"=4215968, "EXPOSURE TIME"=2049184, "CONTRAST GAIN"=3163312, "CONTRAST OFFSET"=3163328, "LIGHT MODE"=2114720, "SENSITIVITY"=2114992, "PHOTON IMAGING MODE"=2115200, "HIGH DYNAMIC RANGE MODE"=3163360, "WHITE BALANCE"=3163568, "TEMPERATURE"=2115232, "TEMPERATURE TARGET"=2115264, "SENSOR COOLER FAN"=2115296, "LINEBUNDLE HEIGHT"=4212192, "MECHANICAL SHUTTER"=2115488, "BACK FOCUS POSITION"=8422304, "TRIGGER CONNECTOR"=1066432, "TRIGGER SOURCE"=1066144, "OUTPUT TRIGGER SOURCE"=1852576, "TRIGGER GLOBAL EXPOSURE"=2049680, "FIRST TRIGGER BEHAVIOR"=2049696, "CHANNEL SYNC"=1852352, "READOUT DIRECTION"=4211904, "PRE HSYNC COUNT"=1852704, "INTERNAL LINE SPEED"=4226000, "INTERNAL LINE INTERVAL"=4226016] ("Parameter")
              w461 = 1 items=["Snap", "Sequence"] ("Capture mode")
              n67 = call "tm_stopcapture.vi"("error in (no error)"=w462, "Handle in"=w465) -> ("error out"=w469:errorcluster, "Handle out"=w470:u32)  [unwired: 8 in]
              n68 = call "tm_unpreparecapture.vi"("error in (no error)"=w469, "Handle in"=w470) -> ("error out"=w455:errorcluster, "Handle out"=w459:u32)  [unwired: 8 in]
              n69 = case shown="2" w456 {
                tunnel: [T9 {"Mode"=1, "Polarity"=2, "Times"=2, "Delay"=0.0} ("Parameters") T9 {"Mode"=2, "Polarity"=2, "Times"=2, "Delay"=0.0} ("Parameters")] -> w457
                frame 1, Default {
                }
                frame 2 {
                }
              }
              n70 = call <userlib>:"tm_setinputtrigger.vi"("error in (no error)"=w455, "Parameters"=w457, "Handle in"=w459) -> ("error out"=w454:errorcluster, "Handle out"=w458:u32)  [unwired: 7 in]
              n71 = call "tm_preparecapture.vi"("error in (no error)"=w454, "Capture mode"=w461, "Handle in"=w458) -> ("error out"=w468:errorcluster, "Buffer Info"=w466:T6, "Handle out"=w467:u32)  [unwired: 5 in, 1 out]
              n72 = call "tm_startcapture_b.vi"("error in (no error)"=w468, "Handle in"=w467) -> ("error out"=w463:errorcluster, "Handle out"=w464:u32)  [unwired: 8 in]
            }
          }
          n73 = local read "stop"() -> (w317:bool)
        }
        n74 = while {
          tunnel: w156 -> [w478]
          shift-right: [w477] -> _
          shift-left: _ -> [w476]
          tunnel: w148 -> [w474]
          stop <- w479 stop-if-true
          n75 = event shown="[1] \"Microscope Settings\": Value Change" {
            selector: _ -> [_ _ _ _ _ _]
            dyn-events: _ -> [_ _ _ _ _ _]
            timeout: 10 -> [_ _ _ _ _ _]
            tunnel: [w480 _ _ _ _ _] -> w479
            tunnel: w478 -> [_ w485 w528 _ _ _]
            tunnel: [_ w482 w525 _ _ w542] -> w477
            tunnel: w476 -> [_ _ w525 _ w535 _]
            tunnel: [_ _ w524 _ w534 _] -> _
            tunnel: w474 -> [_ w481 w524 _ w533 _]
            event "stop": Value Change {
              n76 = event-data() -> ()  [unwired: 1 in, 6 out]
              n77 = local read "stop"() -> (w480:bool)
            }
            event Value Change {
              # "Live video for Calibration and 2D\nScan Modes.\n\nIdle Video for MultiD Scan modes\nUNTIL Begin Scan Button pressed?\n\nMultiD is waiting for trigger"
              n78 = event-data() -> ("NewVal"=w484:T1)  [unwired: 1 in, 5 out]
              n79 = Unbundle By Name(w484) -> ("Mode"=w483:enum16{"X", "XY", "XYZ", "XYZT", "XYZC"})
              n80 = case shown="\"XY\"" w483 {
                tunnel: w485 -> [w494 w511 w520 _ _]
                tunnel: w484 -> [w488 w503 w514 w522 w523]
                tunnel: [w488 w503 w514 w522 w523] -> w482
                tunnel: w481 -> [w487 w502 _ _ _]
                frame "X" {
                  w490 = ModeEnum."generateWaves"  # Mode
                  w491 = 0 ("timeout in ms (-1)")
                  w486 = 1.0 items=["Internal"=1.0, "External"=2.0] ("Trigger Source")
                  n81 = property on="Trigger Source" class="Ring (strict)"("Value"=w486) -> ()  [unwired: 2 in, 2 out]
                  n82 = Bundle("Enum"=CameraControlTypeDef."Trigger Source", "Trigger Source"=w486, "timeout in ms (-1)"=w491) -> (w493:T16)  [unwired: 1 in]
                  n83 = Enqueue Element(queue=w494, element=w493) -> (queue out=w492:refnum<queue>)  [unwired: 2 in, 2 out]
                  n84 = disable-structure shown="Disabled" {
                    disable-tunnel: w492 -> [w499 _]
                    disable-tunnel: w491 -> [w497 _]
                    disable-tunnel: w486 -> [w496 _]
                    frame Disabled {
                      n85 = Bundle("Enum"=CameraControlTypeDef."Preview", "Trigger Source"=w496, "timeout in ms (-1)"=w497) -> (w500:T16)  [unwired: 1 in]
                      n86 = Enqueue Element(queue=w499, element=w500) -> ()  [unwired: 2 in, 3 out]
                    }
                    frame Enabled {
                    }
                  }
                  n87 = Bundle("Mode"=w490, "NewVal"=w488) -> (w489:cluster{"Mode":T8, "NewVal":T1})  [unwired: 1 in]
                  n88 = Enqueue Element(queue=w487, element=w489) -> ()  [unwired: 2 in, 3 out]
                }
                frame "XY" {
                  w505 = ModeEnum."generateWaves"  # Mode
                  w506 = 0 ("timeout in ms (-1)")
                  w501 = 2.0 items=["Internal"=1.0, "External"=2.0] ("Trigger Source")
                  n89 = property on="Trigger Source" class="Ring (strict)"("Value"=w501) -> ()  [unwired: 2 in, 2 out]
                  n90 = Bundle("Enum"=CameraControlTypeDef."Trigger Source", "Trigger Source"=w501, "timeout in ms (-1)"=w506) -> (w510:T16)  [unwired: 1 in]
                  n91 = Enqueue Element(queue=w511, element=w510) -> (queue out=w507:refnum<queue>)  [unwired: 2 in, 2 out]
                  n92 = Bundle("Mode"=w505, "NewVal"=w503) -> (w504:cluster{"Mode":T8, "NewVal":T1})  [unwired: 1 in]
                  n93 = Bundle("Enum"=CameraControlTypeDef."Preview", "Trigger Source"=w501, "timeout in ms (-1)"=w506) -> (w509:T16)  [unwired: 1 in]
                  n94 = Enqueue Element(queue=w502, element=w504) -> ()  [unwired: 2 in, 3 out]
                  n95 = Enqueue Element(queue=w507, element=w509) -> ()  [unwired: 2 in, 3 out]
                }
                frame "XYZ" {
                  w515 = 0 ("timeout in ms (-1)")
                  w513 = 1.0 items=["Internal"=1.0, "External"=2.0] ("Trigger Source")
                  n96 = property on="Trigger Source" class="Ring (strict)"("Value"=w513) -> ()  [unwired: 2 in, 2 out]
                  n97 = Bundle("Enum"=CameraControlTypeDef."Trigger Source", "Trigger Source"=w513, "timeout in ms (-1)"=w515) -> (w519:T16)  [unwired: 1 in]
                  n98 = Enqueue Element(queue=w520, element=w519) -> (queue out=w518:refnum<queue>)  [unwired: 2 in, 2 out]
                  n99 = Bundle("Enum"=CameraControlTypeDef."Idle", "Trigger Source"=w513, "timeout in ms (-1)"=w515) -> (w517:T16)  [unwired: 1 in]
                  n100 = Enqueue Element(queue=w518, element=w517) -> ()  [unwired: 2 in, 3 out]
                }
                frame "XYZT" {
                }
                frame "XYZC" {
                }
              }
            }
            event Value Change {
              w529 = 1.0 items=["Internal"=1.0, "External"=2.0] ("Trigger Source")
              n101 = event-data() -> ()  [unwired: 1 in, 6 out]
              n102 = Bundle("Enum"=CameraControlTypeDef."Readout Mode", "Trigger Source"=w529, "Property ID"=u32 12) -> (w527:T17)  [unwired: 1 in]
              n103 = Enqueue Element(queue=w528, element=w527) -> ()  [unwired: 2 in, 3 out]
            }
            event "Signals Debugger": Value Change {
              n104 = event-data() -> ()  [unwired: 1 in, 6 out]
              n105 = control-ref of="Mixed Signal Graph"() -> (w531:refnum<vi>)
              n106 = call "PopOutGraph.vi"("Mixed Signal Graph 2"=w531) -> ()
            }
            event "Scan": Value Change {
              n107 = event-data() -> ("NewVal"=w532:bool)  [unwired: 1 in, 5 out]
              n108 = case shown="True" w532 {
                tunnel: w535 -> [_ w541]
                tunnel: [w536 w540] -> w534
                tunnel: w533 -> [w536 w539]
                frame False {
                }
                frame True {
                  w538 = ModeEnum."runWaves"  # Mode
                  n109 = Bundle("Mode"=w538, "Value"=w541) -> (w537:cluster{"Mode":T8, "Value":T1})  [unwired: 1 in]
                  n110 = Enqueue Element(queue=w539, element=w537) -> (queue out=w540:refnum<queue>)  [unwired: 2 in, 2 out]
                }
              }
            }
            event Timeout {
              n111 = event-data() -> ()  [unwired: 1 in, 3 out]
              n112 = property on="Microscope Settings" class="Clust (strict)"() -> ("Value"=w542:T1)  [unwired: 2 in, 2 out]
            }
          }
        }
        n113 = while {
          tunnel: w148 -> [w190]
          shift-right: [w185] -> _
          shift-left: _ -> [w184]
          tunnel: w155 -> [w183]
          shift-right: [w179] -> w149
          shift-left: w152 -> [w178]
          shift-right: [w182] -> _
          shift-left: w154 -> [w181]
          shift-right: [w177] -> w150
          shift-left: w151 -> [w176]
          tunnel: [w175] -> w147
          shift-right: [w173] -> w146
          shift-left: _ -> [w172]
          i -> [w174]
          stop <- w189 stop-if-true
          n114 = Dequeue Element(queue=w190, timeout in ms (-1)=1) -> (queue out=w175:refnum<queue>, element=w188:cluster{"Mode":T8, "Microscope Settings":T1})  [unwired: 1 in, 2 out]
          n115 = Unbundle(w188) -> ("Mode"=w187:T8, "Microscope Settings"=w186:T1)
          n116 = case shown="\"generateWaves\"" w187 {
            tunnel: [_ _ _ TRUE] -> w189
            tunnel: w186 -> [_ w206 w270 _]
            tunnel: [w195 w207 w269 w291] -> w185
            tunnel: w184 -> [w195 w198 w269 w291]
            tunnel: w183 -> [_ _ _ _]
            tunnel: w175 -> [_ w197 w271 _]
            tunnel: [w192 w202 w248 w290] -> w177
            tunnel: [w193 w200 w264 w289] -> w179
            tunnel: w178 -> [w193 w199 w272 w289]
            tunnel: [w194 w205 w250 w288] -> w182
            tunnel: w181 -> [w194 w204 w250 w288]
            tunnel: w176 -> [w192 w203 w259 w290]
            tunnel: [w191 w196 w245 w286] -> w173
            tunnel: w172 -> [w191 w196 w244 w286]
            frame "Idle", Default {
            }
            frame "generateWaves" {
              n117 = Unbundle By Name(w206) -> ("Mode"=w201:enum16{"X", "XY", "XYZ", "XYZT", "XYZC"})
              n118 = case shown="\"XY\"" w201 {
                tunnel: [w212 w226] -> w207
                tunnel: w206 -> [_ w232]
                tunnel: [w210 w217] -> w205
                tunnel: w204 -> [w210 _]
                tunnel: w203 -> [w211 w234]
                tunnel: [w211 w234] -> w202
                tunnel: [w208 w233] -> w200
                tunnel: w199 -> [w209 w233]
                tunnel: w198 -> [w212 _]
                tunnel: w197 -> [_ _]
                frame "X", Default {
                  n119 = call "Calibration.vi"("Analogue In"=w209) -> ("Analogue In Out"=w208:refnum<k21>)
                }
                frame "XY" {
                  # "XY Mirrors"
                  n120 = Unbundle(w232) -> ("Piezo Position /um"=w237:dbl, "Exposure/ms"=w235:dbl, "Samples per millisecond"=w229:dbl, "Relax/ms"=w236:dbl, "Camera Delay"=w214:dbl)  [unwired: 4 out]
                  n121 = call "XY Galvo With Homography.vi"("Exposure (ms)"=w235, "Camera Delay /ms"=w214, "Samples /Millisecond"=w229, "Relax (ms)"=w236, "Piezo Position (um)"=w237) -> ("Scan Mirror Signal"=w241:dbl[], "Piezo Signal"=w231:dbl[], "Camera Signal"=w219:dbl[], "Laser Signal"=w224:dbl[], "Z Mirror Signal"=w240:dbl[])  [unwired: 10 in]
                  n122 = Divide(x=0.001 ("y"), y=w229) -> (x/y=w218:dbl)
                  n123 = Bundle By Name("Y"=w241, "dt"=w218) -> (w238:waveform(dbl))  [unwired: 1 in]
                  n124 = Bundle By Name("Y"=w231, "dt"=w218) -> (w230:waveform(dbl))  [unwired: 1 in]
                  n125 = Bundle By Name("Y"=w240, "dt"=w218) -> (w239:waveform(dbl))  [unwired: 1 in]
                  n126 = Build Array(w219) -> (w220:dbl[][])
                  n127 = Build Array(w224) -> (w227:dbl[][])
                  n128 = Transpose 2D Array(2D array=w220) -> (transposed array=w222:dbl[][])
                  n129 = Transpose 2D Array(2D array=w227) -> (transposed array=w223:dbl[][])
                  n130 = Bundle By Name("data"=w222) -> (w221:digitaldata)  [unwired: 1 in]
                  n131 = Bundle By Name("data"=w223) -> (w225:digitaldata)  [unwired: 1 in]
                  n132 = Bundle By Name("Y"=w221, "dt"=w218) -> (w216:digitalwaveform)  [unwired: 1 in]
                  n133 = Bundle By Name("Y"=w225, "dt"=w218) -> (w215:digitalwaveform)  [unwired: 1 in]
                  n134 = Build Array(w238, w239, w230) -> (w226:waveform(dbl)[])
                  n135 = Build Array(w216, w215) -> (w217:digitalwaveform[])
                  n136 = Bundle(w226, "Digital Waveform"=w216, "Digital Waveform"=w215) -> (→"Mixed Signal Graph":T3)  [unwired: 1 in]
                }
              }
            }
            frame "runWaves" {
              n137 = Unbundle By Name(w270) -> ("Samples per millisecond"=w263:dbl)  [unwired: 3 out]
              n138 = Multiply(x=w263, y=1000.0) -> (x*y=w261:dbl)
              n139 = Index Array(array=w269, index=0) -> (element=w267:waveform(dbl))
              n140 = local read "Scan Continuously"() -> (w262:bool)
              n141 = call-poly <vilib>:"Number of Waveform Samples.vi"("waveform in"=w267) -> ("number of samples"=w242:i32)  [unwired: 8 in, 2 out]
              n142 = call-poly <vilib>:"DAQmx Timing.vi"("task/channels in"=w272, "samples per channel"=w242, "rate"=w261, "error in"=w244) -> ("task out"=w275:refnum<k21>, "error out"=w266:errorcluster)  [unwired: 10 in]
              n143 = call-poly <vilib>:"DAQmx Timing.vi"("task/channels in"=w259, "samples per channel"=w242, "rate"=w261, "error in"=w244) -> ("task out"=w260:refnum<k21>, "error out"=w257:errorcluster)  [unwired: 10 in]
              n144 = call-poly <vilib>:"DAQmx Write.vi"("task/channels in"=w275, "data"=w269, "error in"=w266) -> ("task out"=w252:refnum<k21>, "error out"=w255:errorcluster)  [unwired: 10 in, 1 out]
              n145 = call-poly <vilib>:"DAQmx Write.vi"("task/channels in"=w260, "data"=w250, "error in"=w257) -> ("task out"=w251:refnum<k21>, "error out"=w254:errorcluster)  [unwired: 10 in, 1 out]
              n146 = case shown="True" w262 {
                tunnel: w271 -> [w277 w285]
                tunnel: [w278 w284] -> _
                tunnel: w270 -> [w279 w283]
                frame False {
                  n147 = Bundle("Mode"=ModeEnum."Idle", "Microscope Settings"=w279) -> (w280:cluster{"Mode":T8, "Microscope Settings":T1})  [unwired: 1 in]
                  n148 = Enqueue Element(queue=w277, element=w280) -> (queue out=w278:refnum<queue>)  [unwired: 2 in, 2 out]
                }
                frame True {
                  n149 = Bundle("Mode"=ModeEnum."runWaves", "Microscope Settings"=w283) -> (w282:cluster{"Mode":T8, "Microscope Settings":T1})  [unwired: 1 in]
                  n150 = Enqueue Element(queue=w285, element=w282) -> (queue out=w284:refnum<queue>)  [unwired: 2 in, 2 out]
                }
              }
              n151 = Merge Errors(w255, w254) -> (w253:errorcluster)
              n152 = call <vilib>:"DAQmx Start Task.vi"("task/channels in"=w252, "error in"=w253) -> ("task out"=w274:refnum<k21>, "error out"=w273:errorcluster)  [unwired: 12 in]
              n153 = call <vilib>:"DAQmx Start Task.vi"("task/channels in"=w251, "error in"=w253) -> ("task out"=w258:refnum<k21>, "error out"=w256:errorcluster)  [unwired: 12 in]
              n154 = call <vilib>:"DAQmx Wait Until Done.vi"("task/channels in"=w274, "error in"=w273) -> ("task out"=w265:refnum<k21>, "error out"=w247:errorcluster)  [unwired: 12 in]
              n155 = call <vilib>:"DAQmx Wait Until Done.vi"("task/channels in"=w258, "error in"=w256) -> ("task out"=w249:refnum<k21>, "error out"=w246:errorcluster)  [unwired: 12 in]
              n156 = Merge Errors(w247, w246) -> (w245:errorcluster)
              n157 = call <vilib>:"DAQmx Stop Task.vi"("task/channels in"=w249) -> ("task out"=w248:refnum<k21>)  [unwired: 13 in, 1 out]
              n158 = call <vilib>:"DAQmx Stop Task.vi"("task/channels in"=w265) -> ("task out"=w264:refnum<k21>)  [unwired: 13 in, 1 out]
            }
            frame "stop" {
            }
          }
          "Numeric 3" <- w174
        }
        n159 = Merge Errors(w167, w168, w146) -> (w169:errorcluster)
      }
      frame "deinit" {
        n160 = call <vilib>:"DAQmx Stop Task.vi"("task/channels in"=w553) -> ("task out"=w554:refnum<k21>)  [unwired: 13 in, 1 out]
        n161 = call <vilib>:"DAQmx Stop Task.vi"("task/channels in"=w555) -> ("task out"=w556:refnum<k21>)  [unwired: 13 in, 1 out]
        n162 = call <vilib>:"DAQmx Clear Task.vi"("task in"=w554) -> ("error out"=w550:errorcluster)  [unwired: 14 in]
        n163 = call "tm_stopcapture.vi"("error in (no error)"=w565, "Handle in"=w561) -> ("error out"=w568:errorcluster, "Handle out"=w567:u32)  [unwired: 8 in]
        n164 = call <vilib>:"DAQmx Clear Task.vi"("task in"=w556) -> ("error out"=w551:errorcluster)  [unwired: 14 in]
        n165 = call "tm_unpreparecapture.vi"("error in (no error)"=w568, "Handle in"=w567) -> ("error out"=w569:errorcluster, "Handle out"=w566:u32)  [unwired: 8 in]
        n166 = call "tm_closecamera.vi"("error in (no error)"=w569, "Handle in"=w566) -> ("error out"=w570:errorcluster)  [unwired: 9 in]
        n167 = Flush Queue(queue=w543) -> (queue out=w549:refnum<queue>)  [unwired: 1 in, 2 out]
        n168 = call "tm_deinitialize.vi"("error in (no error)"=w570) -> ("error out"=w546:errorcluster)  [unwired: 10 in]
        n169 = Release Queue(queue=w544, error in (no error)=w546) -> (error out=w563:errorcluster)  [unwired: 1 in, 2 out]
        n170 = Release Queue(queue=w549) -> (error out=w552:errorcluster)  [unwired: 2 in, 2 out]
        n171 = Flush Queue(queue=w548, error in (no error)=w546) -> (queue out=w547:refnum<queue>, error out=w545:errorcluster)  [unwired: 1 out]
        n172 = Release Queue(queue=w547, error in (no error)=w545) -> (error out=w562:errorcluster)  [unwired: 1 in, 2 out]
        n173 = Merge Errors(w563, w562, w552, w551, w550) -> (w564:errorcluster)
      }
    }
    n174 = Or(x="stop", y=w17) -> (x .or. y?=w18:bool)
  }
  "error IO" <- w5
  n175 = disable-structure shown="Enabled" {
    frame Disabled {
      # "Parallise decode buffer"
      n176 = call "tm_startcapture_b.vi"() -> ()  [unwired: 10 in, 2 out]
      n177 = call "tm_waitnextframe.vi"() -> ()  [unwired: 8 in, 4 out]
      n178 = call "tm_getframe_a.vi"() -> ()  [unwired: 7 in, 5 out]
    }
    frame Enabled {
    }
  }
